vi "RomiSim_DIFF_POSE_FGV.vi"(9 "in Sim Pose":T1={"TRANSLATION"={"X"=0.0, "Y"=0.0}, "ROTATION"={"VALUE"=0.0, "COS"=1.0, "SIN"=0.0}} {"ROTATION"."SIN" format="%13.4f"; "ROTATION"."COS" format="%13.4f"; "ROTATION"."VALUE" format="%13.4f"; "TRANSLATION"."Y" format="%14.3f"; "TRANSLATION"."X" format="%14.3f"}, 11 "WRITE":bool) -> (3 "out Sim Pose":T1={"TRANSLATION"={"X"=0.0, "Y"=0.0}, "ROTATION"={"VALUE"=0.0, "COS"=1.0, "SIN"=0.0}} {"ROTATION"."SIN" format="%13.4f"; "ROTATION"."COS" format="%13.4f"; "ROTATION"."VALUE" format="%13.4f"; "TRANSLATION"."Y" format="%14.3f"; "TRANSLATION"."X" format="%14.3f"})   [LabVIEW 2019]
uses:
  <vilib>/Rock Robotics/WPI/ThirdParty/JAS_Junk/TrajLib/TypeDef/POSE2D.ctl
  <vilib>/Rock Robotics/WPI/ThirdParty/JAS_Junk/TrajLib/TypeDef/TRANSLATION2D.ctl
  <vilib>/Rock Robotics/WPI/ThirdParty/JAS_Junk/TrajLib/TypeDef/ROTATION2D.ctl
  <vilib>/Rock Robotics/WPI/ThirdParty/JAS_Junk/TrajLib/Trajectory_Library.lvlib
panel:
  # "This is purposefully \n\nNOT re-entrant."
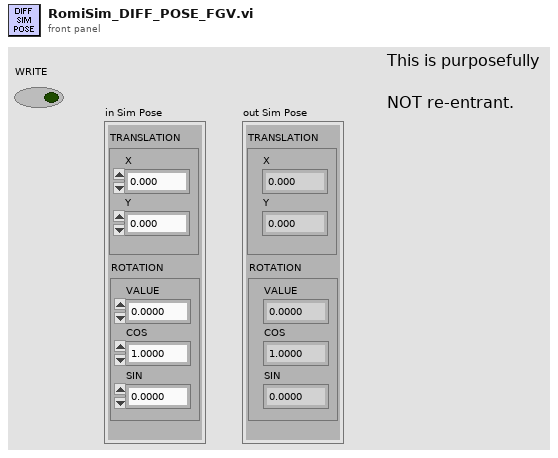
[diagram p1: front panel]
types:
  T1 = typedef "Trajectory_Library.lvlib/POSE2D.ctl" = cluster{"TRANSLATION":T2, "ROTATION":T3}
  T2 = typedef "Trajectory_Library.lvlib/TRANSLATION2D.ctl" = cluster{"X":dbl, "Y":dbl}
  T3 = typedef "Trajectory_Library.lvlib/ROTATION2D.ctl" = cluster{"VALUE":dbl, "COS":dbl, "SIN":dbl}
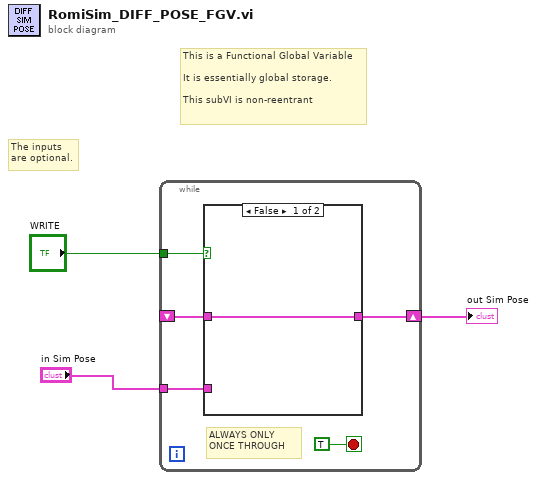
[diagram p0: block diagram]
diagram:
  # "The inputs \nare optional."
  # "This is a Functional Global Variable\n\nIt is essentially global storage.\n\nThis subVI is non-reentrant"
  n1 = while {
    shift-right: [w6] -> w1
    shift-left: _ -> [w4]
    tunnel: "WRITE" -> [w7]
    tunnel: "in Sim Pose" -> [w5]
    stop <- TRUE stop-if-true
    # "ALWAYS ONLY\nONCE THROUGH"
    n2 = case shown="False" w7 {
      tunnel: [w9 w10] -> w6
      tunnel: w5 -> [_ w10]
      tunnel: w4 -> [w9 _]
      frame False {
      }
      frame True {
      }
    }
  }
  "out Sim Pose" <- w1
